vi "Test_step_motor_acc.vi"(0 "Lines":tag="Dev1/port0/line4", 1 "Pulses":i32=50, 3 "error in":errorcluster, 4 "Sample rate":i32=10000) -> (2 "Samples":i64=10000, 5 "error out":errorcluster)   [LabVIEW 2009]
doc: "I. Description:\nThis example demonstrates how to write values to a digital output channel.\n\nII. Instructions for Running:\n1. Select the digital lines on the DAQ device to be written.\n2. Select a value to write.\nNote: The array control is sized for 8 lines, if using a different amount of lines, change the number of elements in the array to equal the number of lines chosen.\n\nIII. Block Diagram Steps:\n1. Create a Digital Output channel. Use one channel for all lines. You can alternatively use one channel for each line, but then use a different polymorphic version of the DAQmx Write VI.\n2. Call the Start VI to start the task.\n3. Write the digital Boolean array data in a loop until the user hits the stop button or an error occurs. This write VI writes a single sample of digital data on demand, so no timeout is necessary.\n4. Call the Clear Task VI to clear the Task.\n5. Use the popup dialog box to display an error or warning if any.\n\nIV. I/O Connections Overview:\nMake sure your signal output terminals match the Lines I/O Control. In this case wire the item to receive the signal to the first eight digital lines on your DAQ Device."
uses:
  <vilib>/DAQmx/configure/timing.llb/DAQmx Timing (Sample Clock).vi
  <vilib>/DAQmx/create/channels.llb/DAQmx Create Channel (DO-Digital Output).vi
  <vilib>/DAQmx/configure/timing.llb/DAQmx Timing (Implicit).vi
  <vilib>/DAQmx/create/channels.llb/DAQmx Create Channel (CO-Pulse Generation-Frequency).vi
  <vilib>/DAQmx/write.llb/DAQmx Write (Digital 1D U8 1Chan NSamp).vi
panel:
  out "stroke":dbl
  out "Freq":dbl
  in  "stop":bool
  in  "Dir":bool
  in  "Motion control card":tag="Dev1"
  in  "Sample Rate":dbl=1000000.0
  out "number of samples written per channel":u32
  # "Channel Parameters"
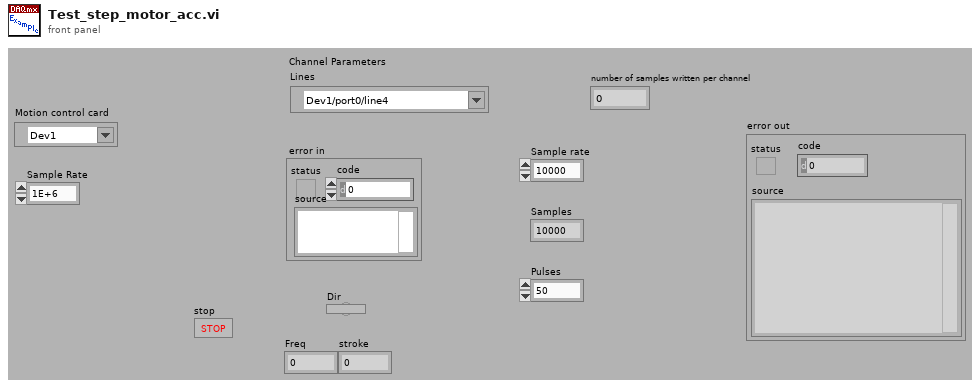
[diagram p1: front panel]
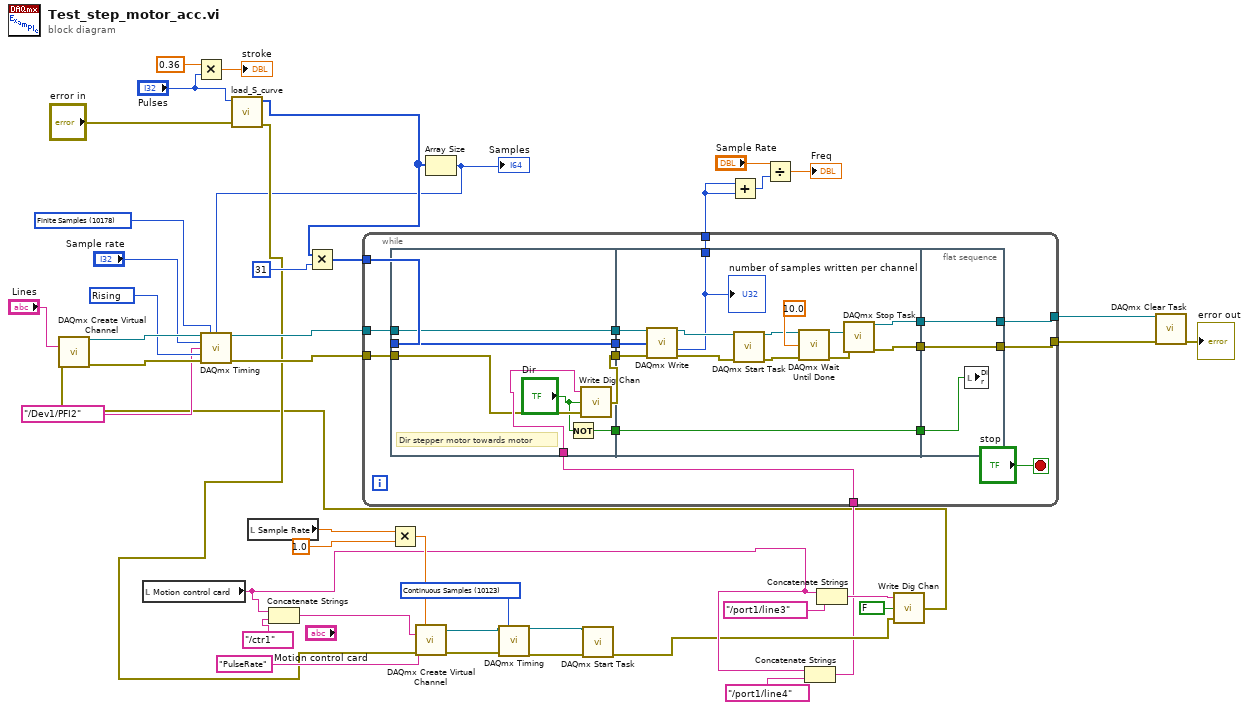
[diagram p0: block diagram]
diagram:
  w32 = 10123 items=["Finite Samples"=10178, "Continuous Samples"=10123, "Hardware Timed Single Point"=12522] ("sample mode")
  w35 = 10280 items=["Rising"=10280, "Falling"=10171] ("active edge")
  w39 = 10178 items=["Finite Samples"=10178, "Continuous Samples"=10123, "Hardware Timed Single Point"=12522] ("sample mode")
  n1 = local read "Motion control card"() -> (w18:tag)
  n2 = Multiply(x=0.36, y="Pulses") -> (x*y=→"stroke":dbl)
  n3 = call "load_S_curve.vi"("error in"="error in", "pulses"="Pulses") -> ("error out"=w12:errorcluster, "S Curve"=w14:u8[])  [unwired: 8 in]
  n4 = local read "Sample Rate"() -> (w28:dbl)
  n5 = Concatenate Strings(w18, tag "/ctr1" ("counter")) -> (w29:string)
  n6 = Multiply(x=w14, y=u8 31 ("Amp")) -> (x*y=w15:u8[])
  n7 = Multiply(x=w28, y=1.0) -> (x*y=w24:dbl)
  n8 = call-poly <vilib>:"DAQmx Create Virtual Channel.vi"("frequency"=w24, "counter"=w29, "name to assign"="PulseRate", "error in"=w12) -> ("task out"=w33:refnum<k21>, "error out"=w23:errorcluster)  [unwired: 5 in, 5 out]
  n9 = Array Size(array=w14) -> (size(s)=w10:i32)
  "Samples" <- w10
  n10 = call-poly <vilib>:"DAQmx Timing.vi"("task/channels in"=w33, "sample mode"=w32, "error in"=w23) -> ("task out"=w26:refnum<k21>, "error out"=w25:errorcluster)  [unwired: 1 in, 10 out]
  n11 = call <vilib>:"DAQmx Start Task.vi"("task/channels in"=w26, "error in"=w25) -> ("error out"=w17:errorcluster)  [unwired: 13 out]
  n12 = Concatenate Strings(w18, tag "/port1/line4" ("Lines")) -> (w9:string)
  n13 = Concatenate Strings(w18, tag "/port1/line3" ("Lines")) -> (w19:string)
  n14 = call "Write Dig Chan.vi"("error in"=w17, "data"=FALSE, "Lines"=w19) -> ("error out"=w8:errorcluster)
  n15 = call-poly <vilib>:"DAQmx Create Virtual Channel.vi"("lines"="Lines", "error in"=w8) -> ("task out"=w42:refnum<k21>, "error out"=w40:errorcluster)  [unwired: 3 in, 9 out]
  n16 = call-poly <vilib>:"DAQmx Timing.vi"("task/channels in"=w42, "sample mode"=w39, "samples per channel"=w10, "rate"="Sample rate", "source"=tag "/Dev1/PFI2", "active edge"=w35, "error in"=w40) -> ("task out"=w41:refnum<k21>, "error out"=w13:errorcluster)  [unwired: 7 out]
  n17 = while {
    tunnel: w41 -> [w52]
    tunnel: [w51] -> w37
    tunnel: [w50] -> w36
    tunnel: w15 -> [w49]
    tunnel: w13 -> [w48]
    tunnel: w9 -> [w47]
    tunnel: [w45] -> w5
    stop <- "stop" stop-if-true
    n18 = flat-sequence {
      tunnel: w48 -> [w63]
      tunnel: w49 -> [w65]
      tunnel: w52 -> [w66]
      tunnel: [w66] -> w59
      tunnel: [w65] -> w58
      tunnel: w47 -> [w64]
      tunnel: [w62] -> w57
      tunnel: [w60] -> w56
      tunnel: w59 -> [w80]
      tunnel: w58 -> [w70]
      tunnel: w57 -> [w69]
      tunnel: [w77] -> w55
      tunnel: [w76] -> w54
      tunnel: [w68] -> w53
      tunnel: w56 -> [w68]
      tunnel: [w67] -> w45
      tunnel: [w82] -> w50
      tunnel: [w83] -> w51
      tunnel: w55 -> [w83]
      tunnel: w54 -> [w82]
      tunnel: w53 -> [w81]
      frame #0 {
        # "Dir stepper motor towards motor"
        n19 = Not(x="Dir") -> (.not. x?=w60:bool)
        n20 = call "Write Dig Chan.vi"("error in"=w63, "data"="Dir", "Lines"=w64) -> ("error out"=w62:errorcluster)
      }
      frame #1 {
        n21 = call-poly <vilib>:"DAQmx Write.vi"("task/channels in"=w80, "data"=w70, "error in"=w69) -> ("task out"=w74:refnum<k21>, "number of samples written per channel"=w67:u32, "error out"=w73:errorcluster)  [unwired: 1 in, 9 out]
        "number of samples written per channel" <- w67
        n22 = call <vilib>:"DAQmx Start Task.vi"("task/channels in"=w74, "error in"=w73) -> ("task out"=w72:refnum<k21>, "error out"=w71:errorcluster)  [unwired: 12 out]
        n23 = call <vilib>:"DAQmx Wait Until Done.vi"("task/channels in"=w72, "timeout (sec)"=10.0, "error in"=w71) -> ("task out"=w79:refnum<k21>, "error out"=w78:errorcluster)  [unwired: 11 out]
        n24 = call <vilib>:"DAQmx Stop Task.vi"("task/channels in"=w79, "error in"=w78) -> ("task out"=w76:refnum<k21>, "error out"=w77:errorcluster)  [unwired: 12 out]
      }
      frame #2 {
        n25 = local write "Dir"(w81) -> ()
      }
    }
  }
  n26 = Add(x=w5, y=w5) -> (x+y=w6:u32)
  n27 = Divide(x="Sample Rate", y=w6) -> (x/y=→"Freq":dbl)
  n28 = call <vilib>:"DAQmx Clear Task.vi"("task in"=w36, "error in"=w37) -> ("error out"=→"error out":errorcluster)  [unwired: 13 out]
